vi "RP compress sweep.vi"(9 "F":dbl[](array[numeric]), 10 "Y":dbl[](array[numeric]), 11 "X":dbl[](array[numeric])) -> (1 "F out":dbl[](array[numeric]), 2 "Y out":dbl[](array[numeric]), 3 "X out":dbl[](array[numeric]))   [LabVIEW 2015]
panel:
  out "Numeric Control":i32
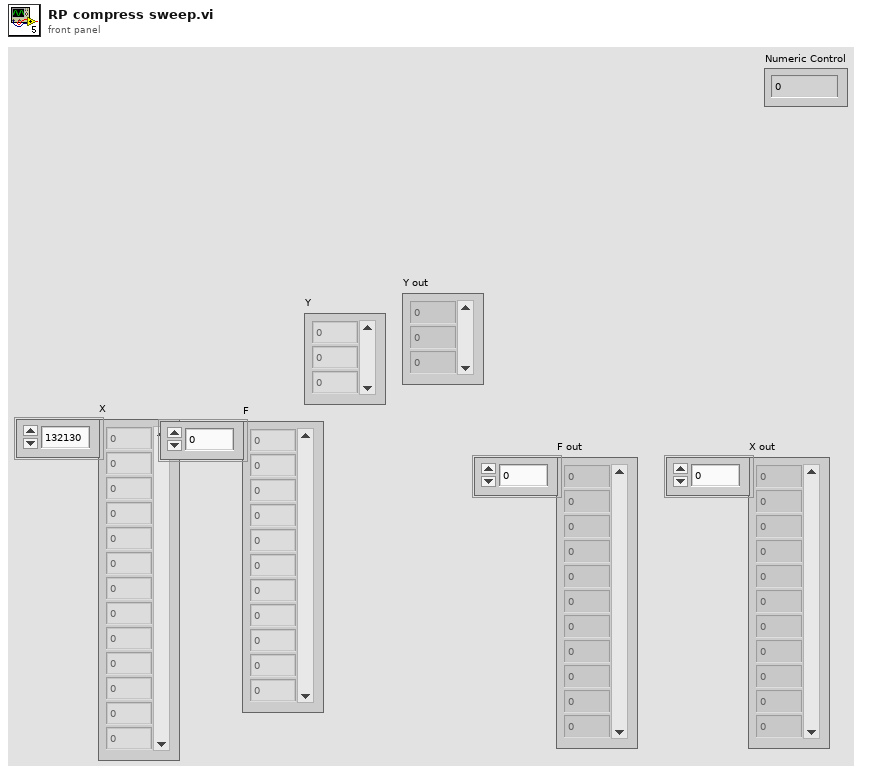
[diagram p1: front panel]
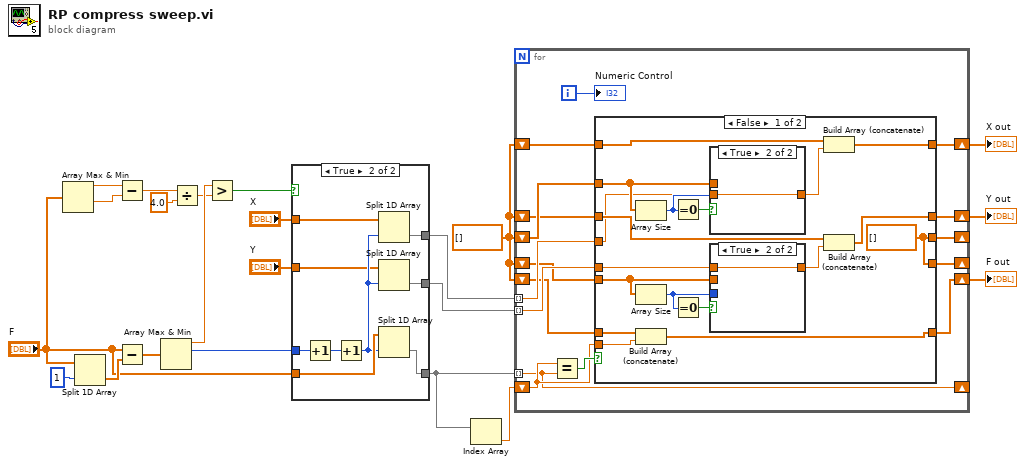
[diagram p0: block diagram]
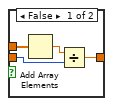
[diagram p3: hidden frame]
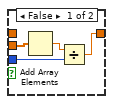
[diagram p4: hidden frame]
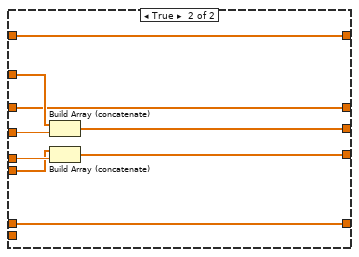
[diagram p5: hidden frame]
diagram:
  w21 = dbl[] [] ("Y")
  n1 = Array Max & Min(array="F") -> (max value=w14:dbl, min value=w13:dbl)  [unwired: 2 out]
  n2 = Split 1D Array(array="F", index=1) -> (second subarray=w16:dbl[])  [unwired: 1 out]
  n3 = Subtract(x=w14, y=w13) -> (x-y=w12:dbl)
  n4 = Subtract(x="F", y=w16) -> (x-y=w15:dbl[])
  n5 = Array Max & Min(array=w15) -> (max value=w10:dbl, max index (indices)=w7:i32)  [unwired: 2 out]
  n6 = Divide(x=w12, y=4.0) -> (x/y=w9:dbl)
  n7 = Greater?(x=w10, y=w9) -> (0:w8:bool)
  n8 = case shown="True" w8 {
    tunnel: w7 -> [_ w34]
    tunnel: "F" -> [w23 w32]
    tunnel: [w23 w31] -> w1
    tunnel: "X" -> [w24 w30]
    tunnel: [w24 w28] -> w4
    tunnel: "Y" -> [w25 w27]
    tunnel: [w25 w26] -> w2
    frame False {
    }
    frame True {
      n9 = Increment(x=w34) -> (x+1=w33:i32)
      n10 = Increment(x=w33) -> (x+1=w29:i32)
      n11 = Split 1D Array(array=w30, index=w29) -> (second subarray=w28:dbl[])  [unwired: 1 out]
      n12 = Split 1D Array(array=w27, index=w29) -> (second subarray=w26:dbl[])  [unwired: 1 out]
      n13 = Split 1D Array(array=w32, index=w29) -> (second subarray=w31:dbl[])  [unwired: 1 out]
    }
  }
  n14 = Index Array(array=w1) -> (element=w22:dbl)  [unwired: 1 in]
  n15 = for {
    tunnel: w1 -> [w36] mode=indexing
    shift-right: [w36] -> _
    shift-left: w22 -> [w38]
    shift-right: [w45] -> _
    shift-left: w21 -> [w47]
    shift-right: [w46] -> _
    shift-left: w21 -> [w50]
    tunnel: w4 -> [w49] mode=indexing
    tunnel: w2 -> [w48] mode=indexing
    shift-right: [w42] -> w20
    shift-left: w21 -> [w43]
    shift-right: [w40] -> w19
    shift-left: w21 -> [w41]
    shift-right: [w37] -> w18
    shift-left: w21 -> [w39]
    i -> [w35]
    n16 = Equal?(x=w38, y=w36) -> (x = y?=w44:bool)
    n17 = case shown="False" w44 {
      tunnel: w50 -> [w54 w87]
      tunnel: w49 -> [w51 w86]
      tunnel: w48 -> [w56 w85]
      tunnel: w47 -> [w67 w84]
      tunnel: [w68 w83] -> w46
      tunnel: [w68 w82] -> w45
      tunnel: w43 -> [w66 w81]
      tunnel: [w65 w81] -> w42
      tunnel: w41 -> [w64 w80]
      tunnel: [w62 w80] -> w40
      tunnel: w39 -> [w61 w79]
      tunnel: w38 -> [w60 _]
      tunnel: [w59 w79] -> w37
      frame False {
        w68 = dbl[] [] ("Y")
        n18 = Array Size(array=w54) -> (size(s)=w52:i32)
        n19 = Array Size(array=w67) -> (size(s)=w58:i32)
        n20 = Build Array (concatenate)(w61, w60) -> (w59:dbl[])
        n21 = Equal To 0?(x=w52) -> (x = 0?=w55:bool)
        n22 = Equal To 0?(x=w58) -> (x = 0?=w57:bool)
        n23 = case shown="True" w55 {
          tunnel: w54 -> [w72 _]
          tunnel: [w70 w73] -> w53
          tunnel: w52 -> [w69 _]
          tunnel: w51 -> [_ w73]
          frame False {
            n24 = Add Array Elements(numeric array=w72) -> (sum=w71:dbl)
            n25 = Divide(x=w71, y=w69) -> (x/y=w70:dbl)
          }
          frame True {
          }
        }
        n26 = case shown="True" w57 {
          tunnel: w67 -> [w77 _]
          tunnel: [w75 w78] -> w63
          tunnel: w58 -> [w74 _]
          tunnel: w56 -> [_ w78]
          frame False {
            n27 = Add Array Elements(numeric array=w77) -> (sum=w76:dbl)
            n28 = Divide(x=w76, y=w74) -> (x/y=w75:dbl)
          }
          frame True {
          }
        }
        n29 = Build Array (concatenate)(w66, w53) -> (w65:dbl[])
        n30 = Build Array (concatenate)(w64, w63) -> (w62:dbl[])
      }
      frame True {
        n31 = Build Array (concatenate)(w87, w86) -> (w83:dbl[])
        n32 = Build Array (concatenate)(w84, w85) -> (w82:dbl[])
      }
    }
    "Numeric Control" <- w35
  }
  "X out" <- w20
  "Y out" <- w19
  "F out" <- w18
